vi "Oddwave Filter_.vi"(10 "Wave Array Input":dbl[][](array[numeric])) -> (2 "x-y":i32, 3 "Averaged Wave Output":dbl[](array[numeric]))   [LabVIEW 2020]
panel:
  out "Averaged Wave":dbl[](array[numeric])
  out "element 2":i32
  out "element":i32
  out "Small":i32
  out "Averaged signals of one pattern 2":dbl[](graph)
  out "Big":i32
  out "Averaged signals of one pattern":dbl[](graph)
  out "Waveform Graph":dbl[][](graph)
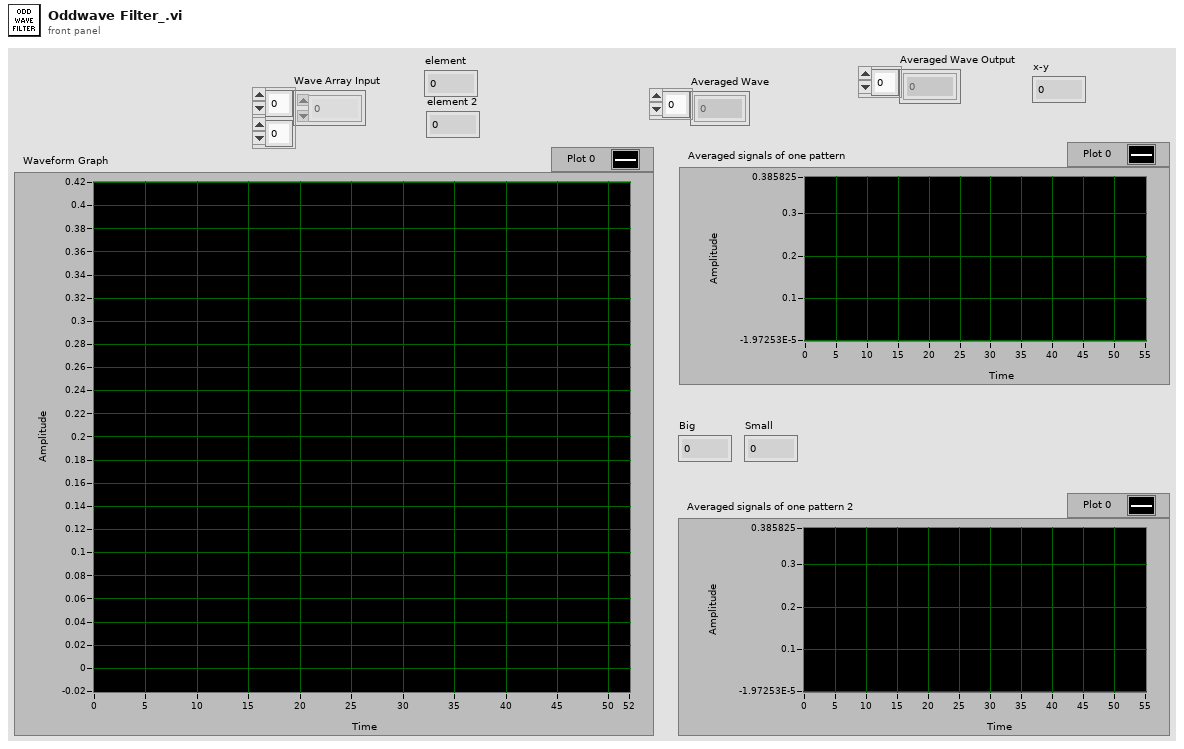
[diagram p1: front panel]
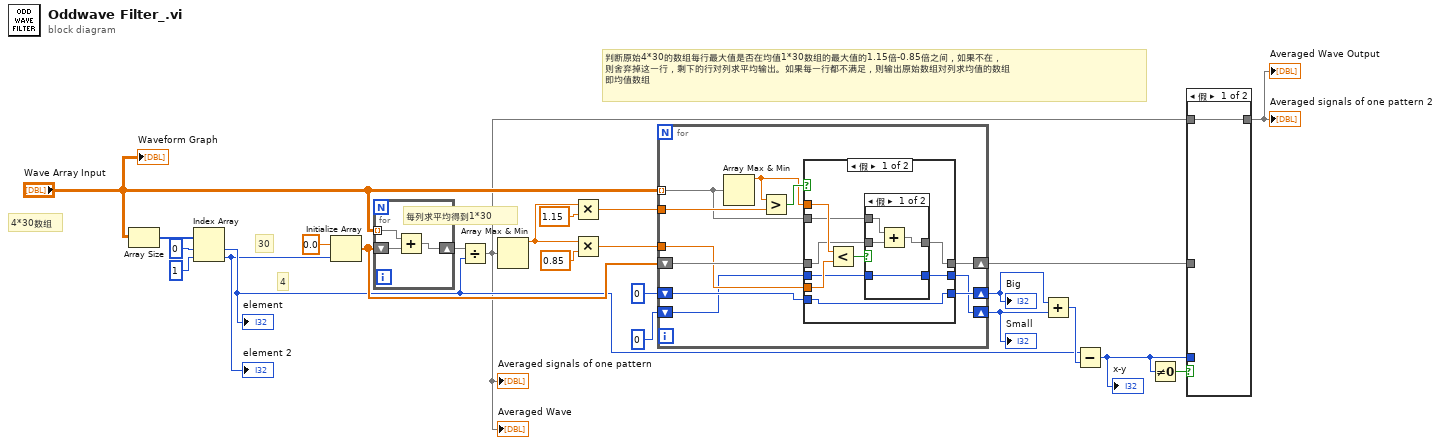
[diagram p0: block diagram]
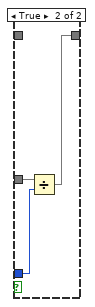
[diagram p2: hidden frame]
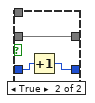
[diagram p3: hidden frame]
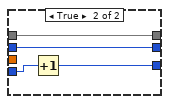
[diagram p4: hidden frame]
diagram:
  # "判断原始4*30的数组每行最大值是否在均值1*30数组的最大值的1.15倍-0.85倍之间，如果不在，\n则舍弃掉这一行，剩下的行对列求平均输出。如果每一行都不满足，则输出原始数组对列求均值的数组\n即均值数组"
  # "每列求平均得到1*30"
  # "30"
  # "4"
  # "4*30数组"
  n1 = Array Size(array="Wave Array Input") -> (size(s)=w10:i32[])
  n2 = Index Array(array=w10, index #1=0 ("index"), index #2=1 ("index")) -> (element #1=w7:i32, element #2=w6:i32)
  "element" <- w7
  "element 2" <- w6
  n3 = Initialize Array(0.0 ("element"), w6) -> (w18:dbl[])
  n4 = for {
    tunnel: "Wave Array Input" -> [w27] mode=indexing
    shift-right: [w26] -> w23
    shift-left: w18 -> [w25]
    n5 = Add(x=w27, y=w25) -> (x+y=w26:dbl[])
  }
  n6 = Divide(x=w23, y=w7) -> (x/y=w2:dbl[])
  "Averaged signals of one pattern" <- w2
  "Averaged Wave" <- w2
  n7 = Array Max & Min(array=w2) -> (max value=w21:dbl)  [unwired: 3 out]
  n8 = Multiply(x=w21, y=1.15) -> (x*y=w19:dbl)
  n9 = Multiply(x=w21, y=0.85) -> (x*y=w17:dbl)
  n10 = for {
    tunnel: "Wave Array Input" -> [w32] mode=indexing
    tunnel: w19 -> [w36]
    shift-right: [w34] -> w15
    shift-left: w18 -> [w35]
    tunnel: w17 -> [w33]
    shift-right: [w30] -> w12
    shift-left: 0 -> [w31]
    shift-right: [w28] -> w13
    shift-left: 0 -> [w29]
    n11 = Array Max & Min(array=w32) -> (max value=w37:dbl)  [unwired: 3 out]
    n12 = Greater?(x=w37, y=w36) -> (0:w38:bool)
    n13 = case shown="假" w38 {
      tunnel: w37 -> [w46 _]
      tunnel: w35 -> [w45 w58]
      tunnel: [w43 w58] -> w34
      tunnel: w33 -> [w44 _]
      tunnel: w32 -> [w42 _]
      tunnel: w31 -> [w41 w57]
      tunnel: [w41 w56] -> w30
      tunnel: [w39 w55] -> w28
      tunnel: w29 -> [w40 w55]
      frame False {
        n14 = Less?(x=w46, y=w44) -> (x < y?=w47:bool)
        n15 = case shown="假" w47 {
          tunnel: w45 -> [w51 w54]
          tunnel: [w49 w54] -> w43
          tunnel: w42 -> [w50 _]
          tunnel: w40 -> [w48 w53]
          tunnel: [w48 w52] -> w39
          frame False {
            n16 = Add(x=w50, y=w51) -> (x+y=w49:dbl[])
          }
          frame True {
            n17 = Increment(x=w53) -> (x+1=w52:i32)
          }
        }
      }
      frame True {
        n18 = Increment(x=w57) -> (x+1=w56:i32)
      }
    }
  }
  "Big" <- w12
  "Small" <- w13
  n19 = Add(x=w12, y=w13) -> (x+y=w11:i32)
  n20 = Subtract(x=w7, y=w11) -> (x-y=w3:i32)
  "x-y" <- w3
  n21 = Not Equal To 0?(x=w3) -> (x != 0?=w4:bool)
  n22 = case shown="假" w4 {
    tunnel: w15 -> [_ w62]
    tunnel: w3 -> [_ w61]
    tunnel: [w59 w60] -> w1
    tunnel: w2 -> [w59 _]
    frame False {
    }
    frame True {
      n23 = Divide(x=w62, y=w61) -> (x/y=w60:dbl[])
    }
  }
  "Averaged signals of one pattern 2" <- w1
  "Averaged Wave Output" <- w1
  "Waveform Graph" <- "Wave Array Input"
